vi "Controller Update Duration.vi"(8 "error in (no error)":errorcluster, 10 "Duration":dbl, 11 "Chef Controller in":refnum<class "Chef Controller.lvclass">) -> (0 "error out":errorcluster, 3 "Chef Controller out":refnum<class "Chef Controller.lvclass">)   [LabVIEW 2024, in "Chef Controller.lvlib" / "Chef Controller.lvclass"]
uses:
  Chef Controller.lvclass
  Chef Controller.lvclass/Chef Controller.ctl
  Chef View Messages/View Update Duration Msg/View Update Duration Msg.lvclass
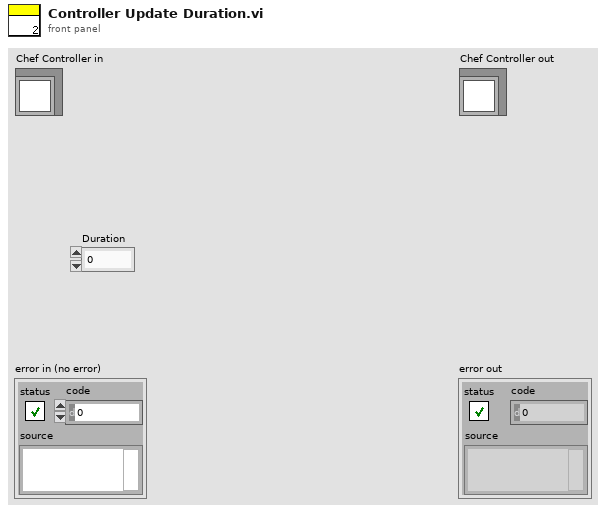
[diagram p1: front panel]
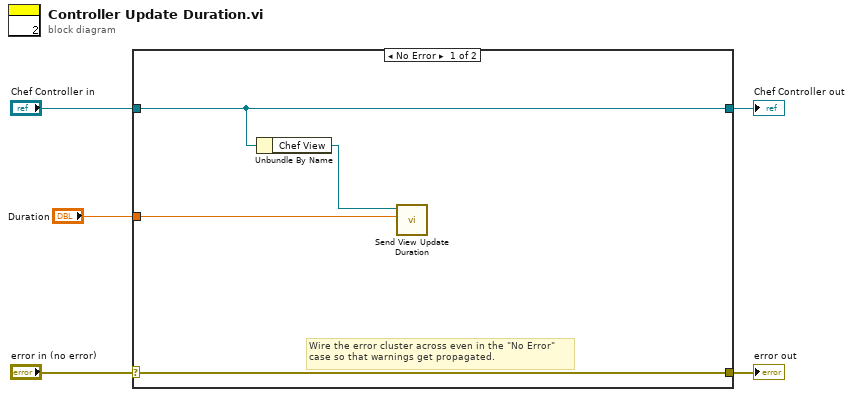
[diagram p0: block diagram]
diagram:
  n1 = case shown="No Error" "error in (no error)" {
    selector: "error in (no error)" -> [w9 w11]
    tunnel: [w9 w11] -> w4
    tunnel: [w8 w10] -> w2
    tunnel: "Chef Controller in" -> [w8 w10]
    tunnel: "Duration" -> [w6 _]
    frame No Error {
      # "Wire the error cluster across even in the \"No Error\"\ncase so that warnings get propagated."
      n2 = Unbundle By Name(w8) -> ("Chef View"=w7:refnum<class "Message Enqueuer.lvclass">)
      n3 = call "Send View Update Duration.vi"("Duration"=w6, "Message Enqueuer"=w7) -> ()  [unwired: 8 in, 2 out]
    }
    frame Error {
    }
  }
  "error out" <- w4
  "Chef Controller out" <- w2
